vi "剪贴板2image.vi"() -> (0 "error out":errorcluster caption="错误输出", 1 "Clipboard has an image?":bool, 3 "Image Out 2":T1(plugin-control))   [LabVIEW 2014]
uses:
  <vilib>/vision/NI_Vision_Development_Module.lvlib
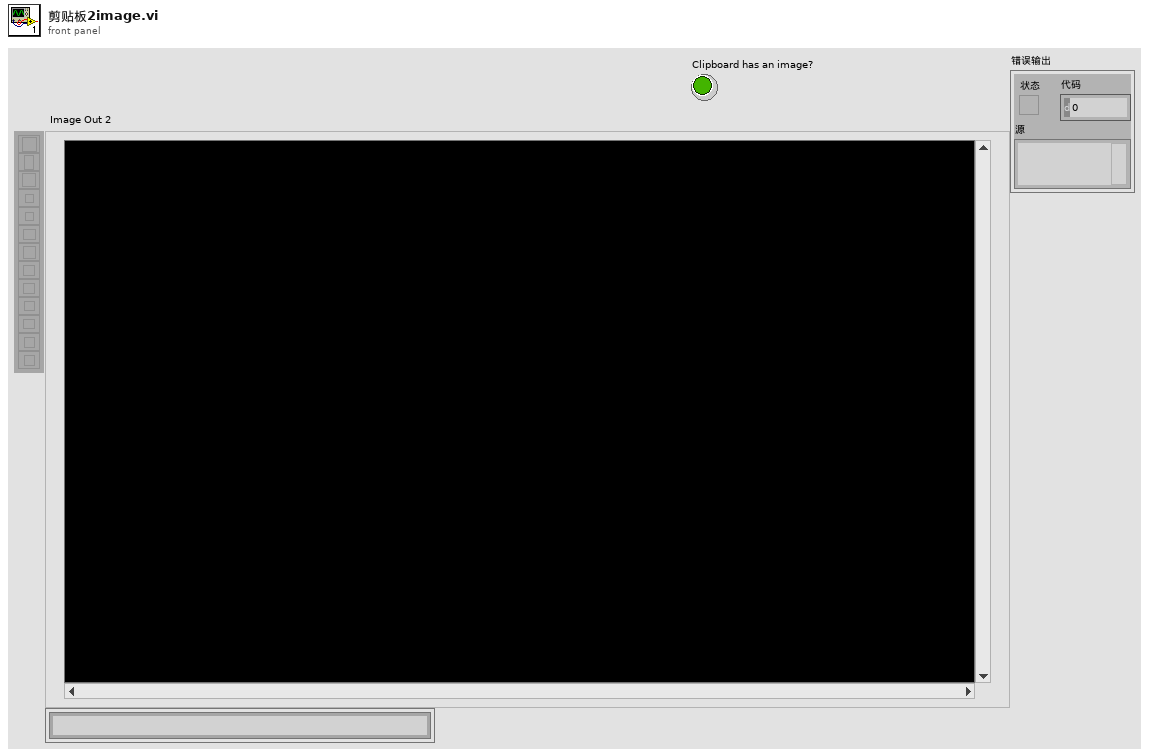
[diagram p1: front panel]
types:
  T1 = typedef "IMAQ Image.ctl" = refnum<image>
  T2 = typedef "Image Type" = u32
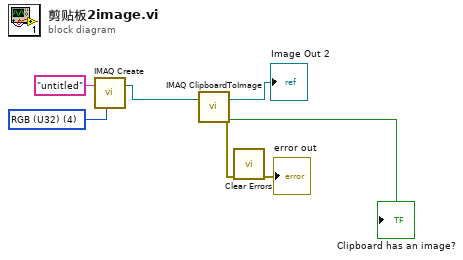
[diagram p0: block diagram]
diagram:
  w4 = T2 4 items=["Grayscale (U8)", "Grayscale (I16)", "Grayscale (SGL)", "Complex (CSG)", "RGB (U32)", "HSL (U32)", "RGB (U64)", "Grayscale (U16)"] ("Image Type")
  n1 = call "IMAQ Create"("Image Name"="untitled", "Image Type"=w4) -> ("New Image"=w7:T1)  [unwired: 3 in, 1 out]
  n2 = call "IMAQ ClipboardToImage"("Image"=w7) -> ("Clipboard has an image?"=→"Clipboard has an image?":bool, "error out"=w2:errorcluster, "Image Out"=→"Image Out 2":T1)  [unwired: 4 in, 1 out]
  n3 = call <vilib>:"Clear Errors.vi"("error in (no error)"=w2) -> ("error out"=→"error out":errorcluster)  [unwired: 1 in, 5 out]
